vi "L16.vi"() -> ()   [LabVIEW 2012]
panel:
  out "sum":i64
  out "String":string
  out "reversed":string
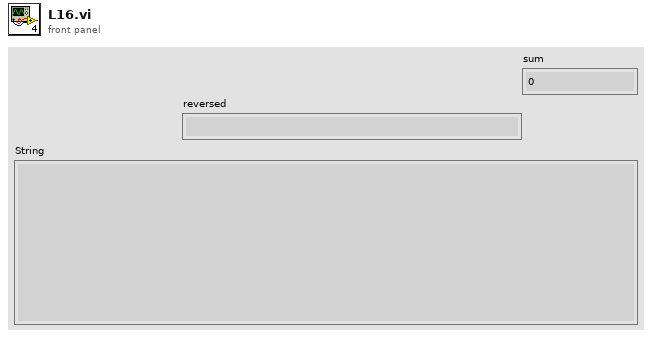
[diagram p1: front panel]
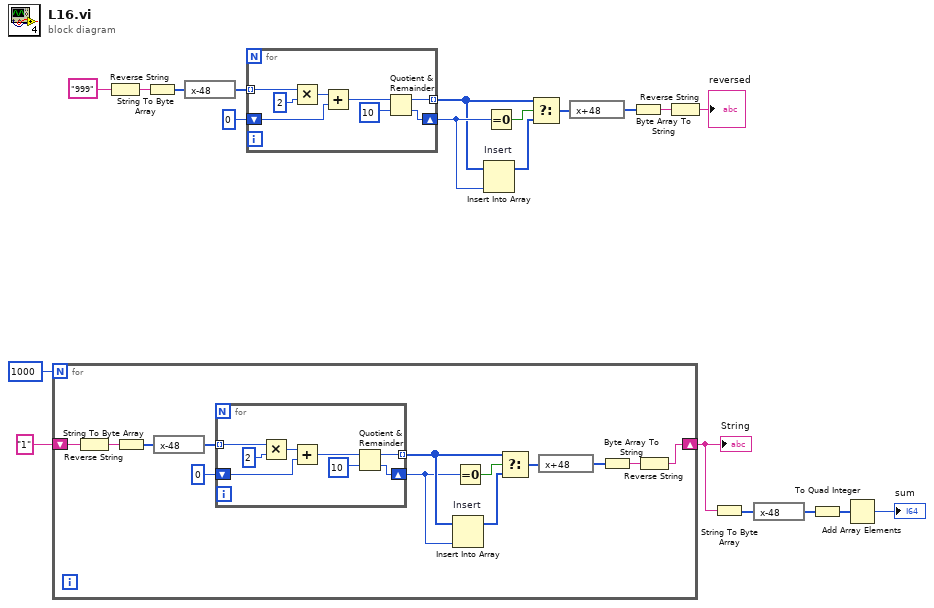
[diagram p0: block diagram]
diagram:
  n1 = for {
    N: 1000 ("Numeric 2") -> [_]
    shift-right: [w21] -> w4
    shift-left: "1" -> [w22]
    n2 = Reverse String(1:w22) -> (0:w23:string)
    n3 = String To Byte Array(string=w23) -> (unsigned byte array=w24:u8[])
    n4 = expression code="x-48"(w24) -> (w25:u8[])
    n5 = for {
      tunnel: w25 -> [w41] mode=indexing
      tunnel: [w38] -> w32 mode=indexing
      shift-right: [w37] -> w29
      shift-left: u8 0 -> [w34]
      n6 = Multiply(x=w41, y=u8 2) -> (x*y=w36:u8)
      n7 = Add(x=w36, y=w34) -> (x+y=w35:u8)
      n8 = Quotient & Remainder(x=w35, y=u8 10) -> (x-y*floor(x/y)=w38:u8, floor(x/y)=w37:u8)
    }
    n9 = Insert Into Array "Insert"(array=w32, new element=w29) -> (w31:u8[])  [unwired: 1 in]
    n10 = Equal To 0?(x=w29) -> (x = 0?=w30:bool)
    n11 = Select(t=w32, s=w30, f=w31) -> (s? t:f=w33:u8[])
    n12 = expression code="x+48"(w33) -> (w27:u8[])
    n13 = Byte Array To String(unsigned byte array=w27) -> (string=w28:string)
    n14 = Reverse String(1:w28) -> (0:w21:string)
  }
  "String" <- w4
  n15 = Reverse String(1:"999") -> (0:w18:string)
  n16 = String To Byte Array(string=w18) -> (unsigned byte array=w17:u8[])
  n17 = expression code="x-48"(w17) -> (w16:u8[])
  n18 = for {
    tunnel: w16 -> [w49] mode=indexing
    tunnel: [w46] -> w8 mode=indexing
    shift-right: [w45] -> w11
    shift-left: u8 0 -> [w42]
    n19 = Multiply(x=w49, y=u8 2) -> (x*y=w44:u8)
    n20 = Add(x=w44, y=w42) -> (x+y=w43:u8)
    n21 = Quotient & Remainder(x=w43, y=u8 10) -> (x-y*floor(x/y)=w46:u8, floor(x/y)=w45:u8)
  }
  n22 = Insert Into Array "Insert"(array=w8, new element=w11) -> (w9:u8[])  [unwired: 1 in]
  n23 = Equal To 0?(x=w11) -> (x = 0?=w10:bool)
  n24 = Select(t=w8, s=w10, f=w9) -> (s? t:f=w7:u8[])
  n25 = expression code="x+48"(w7) -> (w14:u8[])
  n26 = Byte Array To String(unsigned byte array=w14) -> (string=w13:string)
  n27 = Reverse String(1:w13) -> (0:→"reversed":string)
  n28 = String To Byte Array(string=w4) -> (unsigned byte array=w5:u8[])
  n29 = expression code="x-48"(w5) -> (w3:u8[])
  n30 = To Quad Integer(1:w3) -> (0:w2:i64[])
  n31 = Add Array Elements(numeric array=w2) -> (sum=→"sum":i64)
